vi "Protect mode.vi"(9 "ON/OFF":bool, 11 "VISA Source":string) -> (4 "error out":errorcluster)   [LabVIEW 2020]
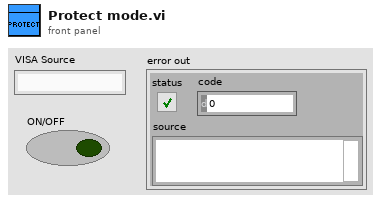
[diagram p1: front panel]
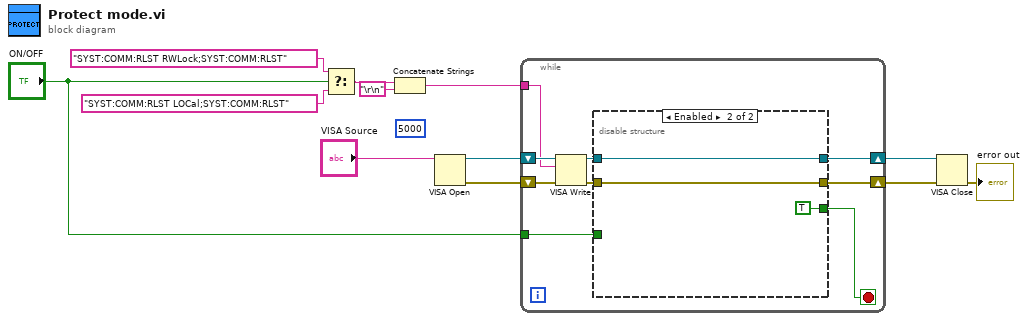
[diagram p0: block diagram]
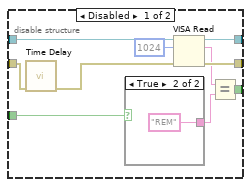
[diagram p2: hidden frame]
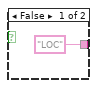
[diagram p3: hidden frame]
diagram:
  (unwired) u32 5000 ("VISA Open timeout (0)")
  n1 = Select(t="SYST:COMM:RLST RWLock;SYST:COMM:RLST" ("string"), s="ON/OFF", f="SYST:COMM:RLST LOCal;SYST:COMM:RLST" ("string")) -> (s? t:f=w5:string)
  n2 = Concatenate Strings(w5, "\r\n") -> (w9:string)
  n3 = VISA Open(VISA resource name="VISA Source") -> (VISA resource name=w12:refnum<visa-resource-name>, error out=w11:errorcluster)  [unwired: 4 in]
  n4 = while {
    tunnel: w9 -> [w19]
    shift-right: [w16] -> w3
    shift-left: w12 -> [w21]
    shift-right: [w17] -> w4
    shift-left: w11 -> [w20]
    tunnel: "ON/OFF" -> [w13]
    stop <- w15 stop-if-true
    n5 = VISA Write(VISA resource name=w21, write buffer=w19, error in (no error)=w20) -> (VISA resource name out=w18:refnum<visa-resource-name>, error out=w14:errorcluster)  [unwired: 1 out]
    n6 = disable-structure shown="Enabled" {
      disable-tunnel: w18 -> [w31 w34]
      disable-tunnel: [w30 _] -> w17
      disable-tunnel: [w29 _] -> w16
      disable-tunnel: [w26 TRUE] -> w15
      disable-tunnel: w14 -> [w25 w35]
      disable-tunnel: w13 -> [w22 _]
      disable-tunnel: [_ w35] -> _
      disable-tunnel: [_ w34] -> _
      frame Disabled {
        n7 = call "Time Delay"("error in (no error)"=w25) -> ("error out"=w24:errorcluster)  [unwired: 10 in]
        n8 = case shown="True" w22 {
          tunnel: ["LOC" ("y") "REM" ("y")] -> w27
          frame False {
          }
          frame True {
          }
        }
        n9 = VISA Read(VISA resource name=w31, byte count=u32 1024, error in (no error)=w24) -> (VISA resource name out=w29:refnum<visa-resource-name>, read buffer=w28:string, error out=w30:errorcluster)  [unwired: 1 out]
        n10 = Equal?(x=w28, y=w27) -> (x = y?=w26:bool)
      }
      frame Enabled {
      }
    }
  }
  n11 = VISA Close(VISA resource name=w3, error in (no error)=w4) -> (error out=→"error out":errorcluster)
